vi "save_mpi_hdf_old.vi"(9 "image dataset":string, 10 "Path":path, 11 "Cluster":T1={"Magnitude meas."=[], "Phase meas."=[], "Shift meas."=[], "cw"=TRUE, "projections per image"=0, "ramp-up readouts"=0, "current sense type"="", "Number of pulses per image"=0, "Rotation enabled"=TRUE, "Rotary position"=[], "Baseline magnitude"=0.0, "Baseline phase"=0.0, "Wait readouts"=0, "Shift waveform type"="", "Shift enabled"=TRUE, "Time domain data"=[], "Motor pulse duration"=0.0, "Shift start"=0.0, "Shift stop"=0.0, "Notes"="", "Reconstructed image"=bytes[0], "Rotary encoder type"="", "Image start"=timestamp(0 s since 1904-01-01), "Image stop"=timestamp(0 s since 1904-01-01), "readouts per projection"=0, "Recon enabled"=FALSE, "Bidirectional shift"=FALSE, "Imager mode"="", "Shift delay"=0.0, "Shift frequency"=0.0, "Image time (calc)"=0.0, "Initial encoder position"=0.0, "Recon data"=[]}) -> ()   [LabVIEW 2019]
uses:
  <vilib>/UPVI/lvhdf5/file.llb/LVH5F Operation.ctl
  <vilib>/Utility/miscctls.llb/LVRectTypeDef.ctl
  <vilib>/UPVI/lvhdf5/group.llb/H5G_obj_t.ctl
  <vilib>/UPVI/lvhdf5/dataset.llb/LVH5D Operation.ctl
  <vilib>/UPVI/lvhdf5/attribute.llb/LVH5A Operation.ctl
  <vilib>/UPVI/lvhdf5/identifier.llb/Not an HDF5 Refnum Constant.vi
  <vilib>/UPVI/lvhdf5/common.llb/To HDF5 Ref.vi
  global_variables.vi
  <vilib>/UPVI/lvhdf5/attribute.llb/Write Multiple Attributes.vi
  <vilib>/UPVI/lvhdf5/utility.llb/Select HDF5 Dialog.vi
  <vilib>/UPVI/lvhdf5/utility.llb/Select HDF5 Dialog (Object Only).vi
  <vilib>/UPVI/lvhdf5/dataset.llb/Simple H5Dwrite (Variant).vi
  <vilib>/UPVI/lvhdf5/dataset.llb/H5Dclose.vi
  <vilib>/UPVI/lvhdf5/attribute.llb/LVH5 Write Attributes.xnode
  <vilib>/UPVI/lvhdf5/library.llb/HDF5 Ref.ctl
  <vilib>/UPVI/lvhdf5/dataset.llb/Simple H5Dwrite.xnode
  <vilib>/UPVI/lvhdf5/dataset.llb/Write Dataset with Attributes.xnode
  <vilib>/Utility/VariantDataType/GetClusterInfo.vi
  <vilib>/Utility/VariantDataType/VariantType.lvlib
  <vilib>/Utility/VariantDataType/GetTypeInfo.vi
  <vilib>/UPVI/lvhdf5/attribute.llb/Cluster to Attribute Array.xnode
  <vilib>/Utility/error.llb/Error Cluster From Error Code.vi
  <vilib>/UPVI/lvhdf5/dataset.llb/OpenCreateReplace Dataset by Element Type.vi
  <vilib>/UPVI/lvhdf5/dataspace.llb/H5Sselect_hyperslab.vi
  <vilib>/UPVI/lvhdf5/dataset.llb/H5Dwrite (Variant).vi
  <vilib>/UPVI/lvhdf5/dataset.llb/H5Dget_space.vi
  <vilib>/UPVI/lvhdf5/attribute.llb/private/LVH5AwriteWDTAttrs.vi
  <vilib>/UPVI/lvhdf5/dataspace.llb/H5Sclose.vi
  <vilib>/UPVI/lvhdf5/utility.llb/Select HDF5 Dialog (File and Object).vi
  <resource>/objmgr/daqmx.rc
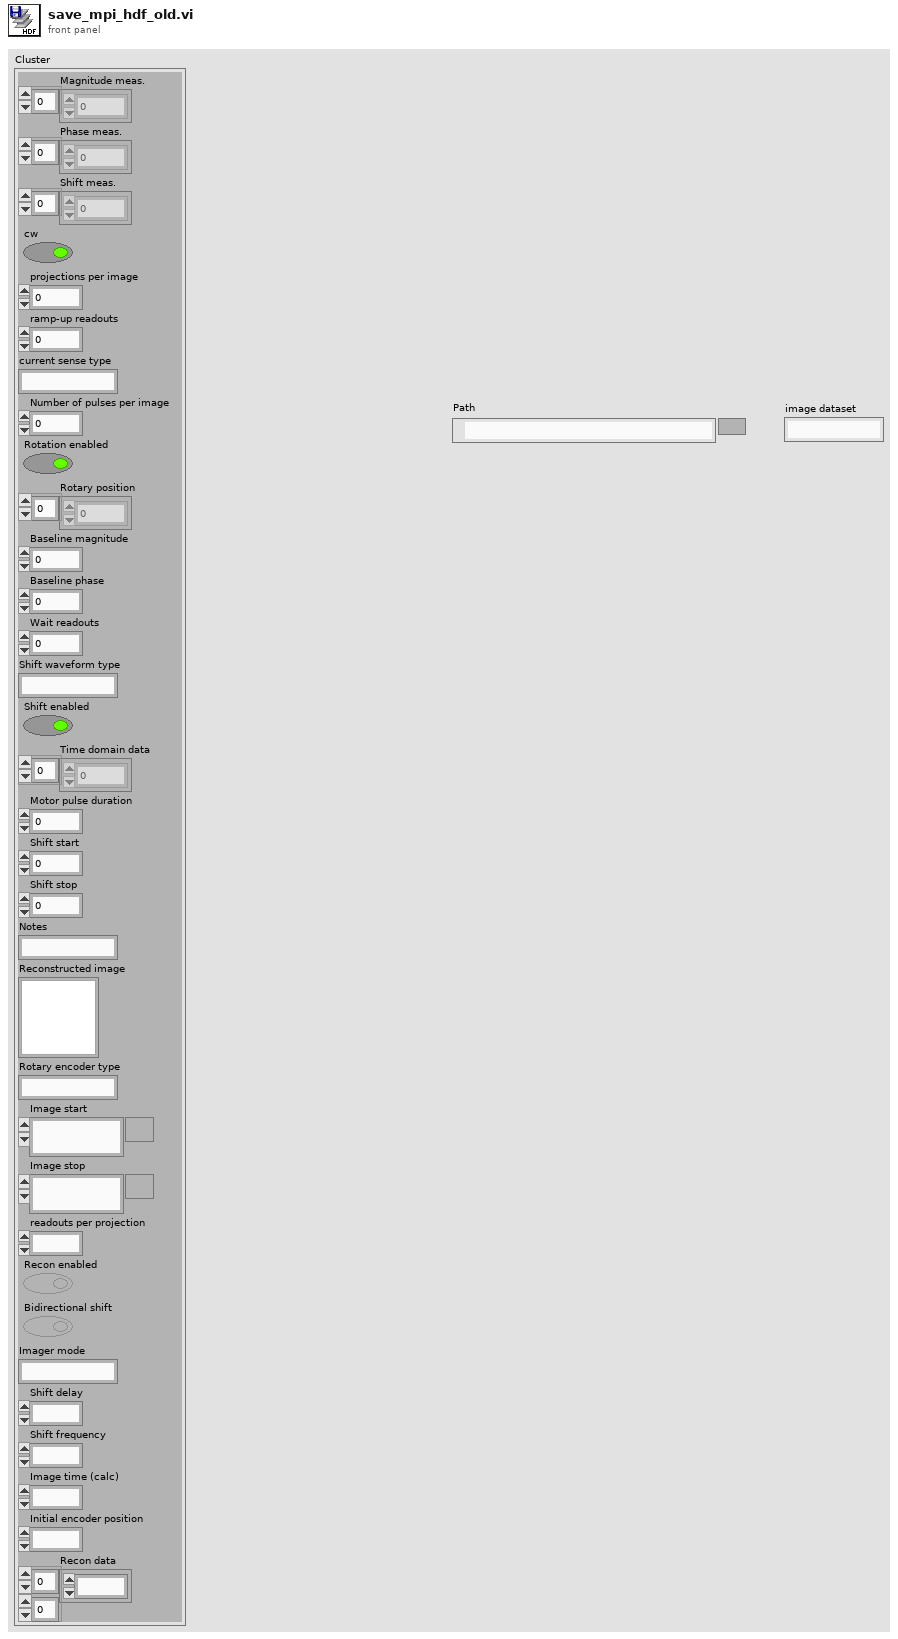
[diagram p1: front panel]
types:
  T1 = cluster{"Magnitude meas.":dbl[], "Phase meas.":dbl[], "Shift meas.":dbl[], "cw":bool, "projections per image":i32, "ramp-up readouts":i32, "current sense type":string, "Number of pulses per image":i32, "Rotation enabled":bool, "Rotary position":dbl[], "Baseline magnitude":dbl, "Baseline phase":dbl, "Wait readouts":i32, "Shift waveform type":string, "Shift enabled":bool, "Time domain data":dbl[], "Motor pulse duration":dbl, "Shift start":dbl, "Shift stop":dbl, "Notes":string, "Reconstructed image":picture, "Rotary encoder type":string, "Image start":timestamp, "Image stop":timestamp, "readouts per projection":i32, "Recon enabled":bool, "Bidirectional shift":bool, "Imager mode":string, "Shift delay":dbl, "Shift frequency":dbl, "Image time (calc)":dbl, "Initial encoder position":dbl, "Recon data":dbl[][]}
  T2 = typedef "LVH5F Operation.ctl" = enum16{"open", "open or create", "create or replace", "create or replace (with confirmation)", "create", "open (read only)"}
  T3 = typedef "HDF5 Ref.ctl" = refnum<k1>
  T4 = typedef "LVH5A Operation.ctl" = enum16{"open", "replace", "create", "open or create", "create or replace", "create or replace with confirmation"}
  T5 = typedef "LVRectTypeDef.ctl" = cluster{"Left":i16, "Top":i16, "Right":i16, "Bottom":i16}
  T6 = cluster{"Behavior":enum32{"Invalid", "Default", "Floating", "Floating/Auto-Hide", "Modal"}, "Position":T5, "Center":bool, "Title":string}
  T7 = typedef "LVH5D Operation.ctl" = enum16{"open", "replace", "create", "open or create", "create or replace", "create or replace with confirmation"}
  T8 = typedef "H5G_obj_t.ctl" = i32
  T9 = cluster{"Object Types (any)":T8[], "Object Pattern":string}
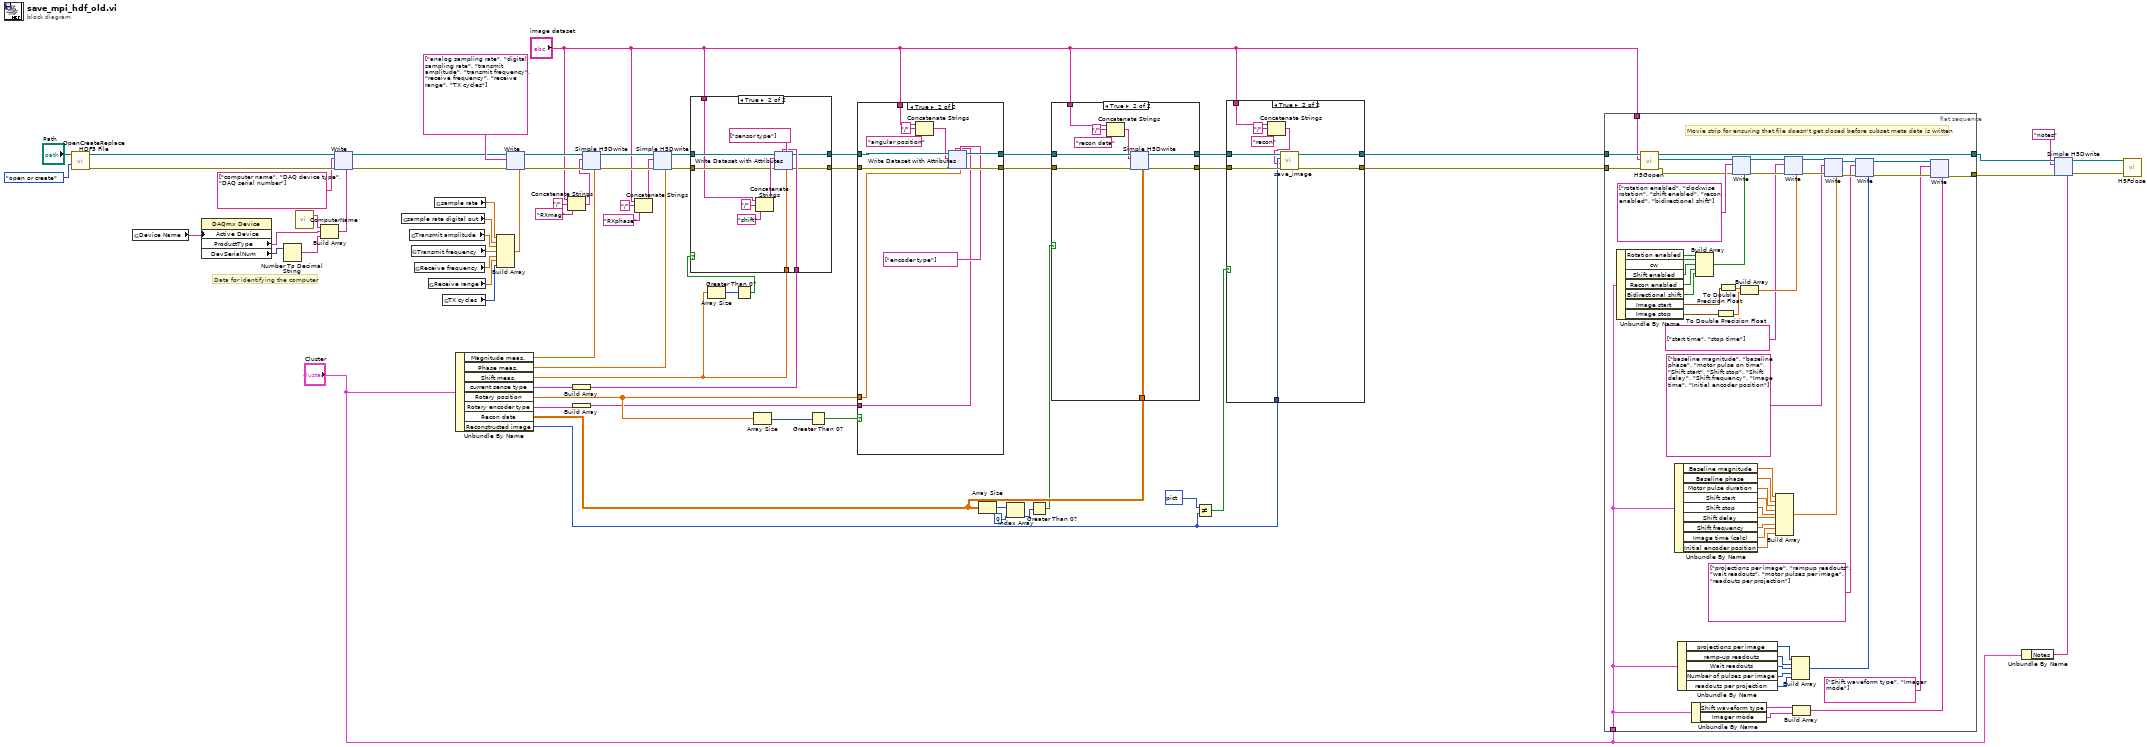
[diagram p0: block diagram]
diagram:
  # "Data for identifying the computer"
  n1 = call <vilib>:"OpenCreateReplace HDF5 File.vi"("function (open or create)"=LVH5F_Operation."open or create", "path"="Path") -> ("error out"=w62:errorcluster, "HDF5 Ref out"=w63:T3)  [unwired: 6 in]
  n2 = global read "global_variables.vi" "Device Name"() -> (w3:tag)
  n3 = property class="DAQmx Device"("Active Device"=w3) -> ("ProductType"=w66:string, "DevSerialNum"=w68:u32)  [unwired: 2 in, 2 out]
  n4 = Number To Decimal String(number=w68) -> (decimal integer string=w67:string)  [unwired: 1 in]
  n5 = call "ComputerName.vi"() -> ("String/Binary data"=w65:string)  [unwired: 4 in, 1 out]
  n6 = Build Array(w65, w66, w67) -> (w64:string[])
  n7 = xnode "Write"("HDF5 Ref"=w63, "error in (no error)"=w62, "Name(s)"=string[] ["computer name", "DAQ device type", "DAQ serial number"], "Value(s)"=w64) -> ("HDF5 Ref out"=w28:T3, "error out"=w27:errorcluster)  [unwired: 1 in]
  n8 = global read "global_variables.vi" "sample rate digital out"() -> (w60:dbl)
  n9 = global read "global_variables.vi" "Transmit amplitude"() -> (w59:dbl)
  n10 = global read "global_variables.vi" "Transmit frequency"() -> (w58:dbl)
  n11 = global read "global_variables.vi" "Receive frequency"() -> (w31:dbl)
  n12 = global read "global_variables.vi" "Receive range"() -> (w30:dbl)
  n13 = global read "global_variables.vi" "sample rate"() -> (w61:dbl)
  n14 = global read "global_variables.vi" "TX cycles"() -> (w29:i32)
  n15 = Unbundle By Name("Cluster") -> ("Magnitude meas."=w49:dbl[], "Phase meas."=w43:dbl[], "Shift meas."=w24:dbl[], "current sense type"=w40:string, "Rotary position"=w35:dbl[], "Rotary encoder type"=w38:string, "Recon data"=w9:dbl[][], "Reconstructed image"=w13:picture)
  n16 = Build Array(w61, w60, w59, w58, w31, w30, w29) -> (w55:dbl[])
  n17 = xnode "Write"("HDF5 Ref"=w28, "error in (no error)"=w27, "Name(s)"=string[] ["analog sampling rate", "digital sampling rate", "transmit amplitude", "transmit frequency", "receive frequency", "receive range", "TX cycles"], "Value(s)"=w55) -> ("HDF5 Ref out"=w52:T3, "error out"=w51:errorcluster)  [unwired: 1 in]
  n18 = Concatenate Strings("image dataset", "/" ("string"), "RXmag" ("string")) -> (w50:string)
  n19 = Build Array(w40) -> (w39:string[])
  n20 = Build Array(w38) -> (w32:string[])
  n21 = xnode "Simple H5Dwrite"("Dataset Path"=w50, "error in (no error)"=w51, "HDF5 Path or Ref"=w52, "Data"=w49) -> ("HDF5 Ref out"=w48:T3, "error out"=w47:errorcluster)  [unwired: 4 in, 1 out]
  n22 = Concatenate Strings("image dataset", "/" ("string"), "RXphase" ("string")) -> (w44:string)
  n23 = xnode "Simple H5Dwrite"("Dataset Path"=w44, "error in (no error)"=w47, "HDF5 Path or Ref"=w48, "Data"=w43) -> ("HDF5 Ref out"=w42:T3, "error out"=w41:errorcluster)  [unwired: 4 in, 1 out]
  n24 = Array Size(array=w24) -> (size(s)=w25:i32)
  n25 = Greater Than 0?(x=w25) -> (x > 0?=w26:bool)
  n26 = case shown="True" w26 {
    tunnel: w42 -> [w72 w80]
    tunnel: w41 -> [w71 w79]
    tunnel: w24 -> [_ w78]
    tunnel: w39 -> [_ w76]
    tunnel: [w72 w75] -> w37
    tunnel: [w71 w74] -> w36
    tunnel: "image dataset" -> [_ w73]
    frame False {
    }
    frame True {
      n27 = Concatenate Strings(w73, "/" ("string"), "shift" ("string")) -> (w83:string)
      n28 = xnode "Write Dataset with Attributes"("Dataset Path"=w83, "error in (no error)"=w79, "HDF5 Path or Ref"=w80, "Attribute Name(s)"=string[] ["sensor type"], "Attribute Value(s)"=w76, "Data"=w78) -> ("HDF5 Ref out"=w75:T3, "error out"=w74:errorcluster)  [unwired: 2 in, 1 out]
    }
  }
  n29 = Array Size(array=w35) -> (size(s)=w34:i32)
  n30 = Greater Than 0?(x=w34) -> (x > 0?=w33:bool)
  n31 = case shown="True" w33 {
    tunnel: w37 -> [w379 w387]
    tunnel: w36 -> [w378 w386]
    tunnel: [w379 w385] -> w19
    tunnel: [w378 w384] -> w18
    tunnel: w35 -> [_ w381]
    tunnel: "image dataset" -> [_ w388]
    tunnel: w32 -> [_ w380]
    frame False {
    }
    frame True {
      n32 = Concatenate Strings(w388, "/" ("string"), "angular position" ("string")) -> (w382:string)
      n33 = xnode "Write Dataset with Attributes"("Dataset Path"=w382, "error in (no error)"=w386, "HDF5 Path or Ref"=w387, "Attribute Name(s)"=string[] ["encoder type"], "Attribute Value(s)"=w380, "Data"=w381) -> ("HDF5 Ref out"=w385:T3, "error out"=w384:errorcluster)  [unwired: 2 in, 1 out]
    }
  }
  n34 = Array Size(array=w9) -> (size(s)=w7:i32[])
  n35 = Index Array(array=w7, index=0) -> (element=w5:i32)
  n36 = Greater Than 0?(x=w5) -> (x > 0?=w4:bool)
  n37 = case shown="True" w4 {
    tunnel: [w686 w695] -> w17
    tunnel: [w685 w694] -> w16
    tunnel: w19 -> [w686 w693]
    tunnel: w18 -> [w685 w692]
    tunnel: "image dataset" -> [_ w688]
    tunnel: w9 -> [_ w687]
    frame False {
    }
    frame True {
      n38 = Concatenate Strings(w688, "/" ("string"), "recon data" ("string")) -> (w689:string)
      n39 = xnode "Simple H5Dwrite"("Dataset Path"=w689, "error in (no error)"=w692, "HDF5 Path or Ref"=w693, "Data"=w687) -> ("HDF5 Ref out"=w695:T3, "error out"=w694:errorcluster)  [unwired: 4 in, 1 out]
    }
  }
  n40 = Not Equal?(x=picture data[5B] ("Reconstructed image"), y=w13) -> (x != y?=w14:bool)
  n41 = case shown="True" w14 {
    tunnel: w17 -> [w899 w908]
    tunnel: [w899 w907] -> w2
    tunnel: [w898 w906] -> w1
    tunnel: w16 -> [w898 w905]
    tunnel: w13 -> [_ w904]
    tunnel: "image dataset" -> [_ w901]
    frame False {
    }
    frame True {
      n42 = Concatenate Strings(w901, "/" ("string"), "recon" ("string")) -> (w900:string)
      n43 = call "save_image.vi"("error in (no error)"=w905, "dset_name"=w900, "picture"=w904, "HDF5 Ref"=w908) -> ("error out"=w906:errorcluster, "HDF5 Ref out"=w907:T3)  [unwired: 6 in]
    }
  }
  n44 = flat-sequence {
    tunnel: w1 -> [w935]
    tunnel: w2 -> [w959]
    tunnel: [w958] -> w23
    tunnel: "Cluster" -> [w920]
    tunnel: "image dataset" -> [w953]
    tunnel: [w921] -> w22
    frame #0 {
      # "Movie strip for ensuring that file doesn't get closed before subset meta data is written"
      n45 = Unbundle By Name(w920) -> ("Rotation enabled"=w957:bool, "cw"=w956:bool, "Shift enabled"=w955:bool, "Recon enabled"=w954:bool, "Bidirectional shift"=w909:bool, "Image start"=w934:timestamp, "Image stop"=w931:timestamp)
      n46 = call <vilib>:"H5Gopen.vi"("error in (no error)"=w935, "Name"=w953, "HDF5 Ref"=w959) -> ("error out"=w949:errorcluster, "HDF5 Group Ref"=w952:T3, "HDF5 Ref out"=w958:T3)  [unwired: 4 in]
      n47 = Unbundle By Name(w920) -> ("Baseline magnitude"=w944:dbl, "Baseline phase"=w943:dbl, "Motor pulse duration"=w938:dbl, "Shift start"=w937:dbl, "Shift stop"=w936:dbl, "Shift delay"=w914:dbl, "Shift frequency"=w913:dbl, "Image time (calc)"=w912:dbl, "Initial encoder position"=w910:dbl)
      n48 = Unbundle By Name(w920) -> ("projections per image"=w927:i32, "ramp-up readouts"=w925:i32, "Wait readouts"=w924:i32, "Number of pulses per image"=w919:i32, "readouts per projection"=w915:i32)
      n49 = Unbundle By Name(w920) -> ("Shift waveform type"=w918:string, "Imager mode"=w911:string)
      n50 = Build Array(w957, w956, w955, w954, w909) -> (w950:bool[])
      n51 = To Double Precision Float(number=w931) -> (double precision float=w932:dbl)
      n52 = To Double Precision Float(number=w934) -> (double precision float=w933:dbl)
      n53 = xnode "Write"("HDF5 Ref"=w952, "error in (no error)"=w949, "Name(s)"=string[] ["rotation enabled", "clockwise rotation", "shift enabled", "recon enabled", "bidirectional shift"], "Value(s)"=w950) -> ("HDF5 Ref out"=w948:T3, "error out"=w947:errorcluster)  [unwired: 1 in]
      n54 = Build Array(w933, w932) -> (w946:dbl[])
      n55 = Build Array(w944, w943, w938, w937, w936, w914, w913, w912, w910) -> (w939:dbl[])
      n56 = xnode "Write"("HDF5 Ref"=w948, "error in (no error)"=w947, "Name(s)"=string[] ["start time", "stop time"], "Value(s)"=w946) -> ("HDF5 Ref out"=w942:T3, "error out"=w941:errorcluster)  [unwired: 1 in]
      n57 = Build Array(w927, w925, w924, w919, w915) -> (w926:i32[])
      n58 = Build Array(w918, w911) -> (w917:string[])
      n59 = xnode "Write"("HDF5 Ref"=w942, "error in (no error)"=w941, "Name(s)"=string[] ["baseline magnitude", "baseline phase", "motor pulse on time", "Shift start", "Shift stop", "Shift delay", "Shift frequency", "Image time", "Initial encoder position"], "Value(s)"=w939) -> ("HDF5 Ref out"=w929:T3, "error out"=w930:errorcluster)  [unwired: 1 in]
      n60 = xnode "Write"("HDF5 Ref"=w929, "error in (no error)"=w930, "Name(s)"=string[] ["projections per image", "rampup readouts", "wait readouts", "motor pulses per image", "readouts per projection"], "Value(s)"=w926) -> ("HDF5 Ref out"=w923:T3, "error out"=w922:errorcluster)  [unwired: 1 in]
      n61 = xnode "Write"("HDF5 Ref"=w923, "error in (no error)"=w922, "Name(s)"=string[] ["Shift waveform type", "Imager mode"], "Value(s)"=w917) -> ("error out"=w921:errorcluster)  [unwired: 1 in, 1 out]
    }
  }
  n62 = Unbundle By Name("Cluster") -> ("Notes"=w20:string)
  n63 = xnode "Simple H5Dwrite"("Dataset Path"="notes", "error in (no error)"=w22, "HDF5 Path or Ref"=w23, "Data"=w20) -> ("HDF5 Ref out"=w11:T3, "error out"=w10:errorcluster)  [unwired: 4 in, 1 out]
  n64 = call <vilib>:"H5Fclose.vi"("error in (no error)"=w10, "HDF5 Ref"=w11) -> ()  [unwired: 7 in, 1 out]
